vi "KundtsTube.vi"() -> ()   [LabVIEW 2015]
panel:
  in  "?":T1
  out "Gain vs Frequency":cluster{"X":dbl, "Y":dbl}[](graph)
  in  "Number of Samples":dbl
  in  "Sampling Rate":dbl
  in  "stop":bool
  out "Waveform Graph":dynamicdata(graph)
  in  "Amplitude":dbl
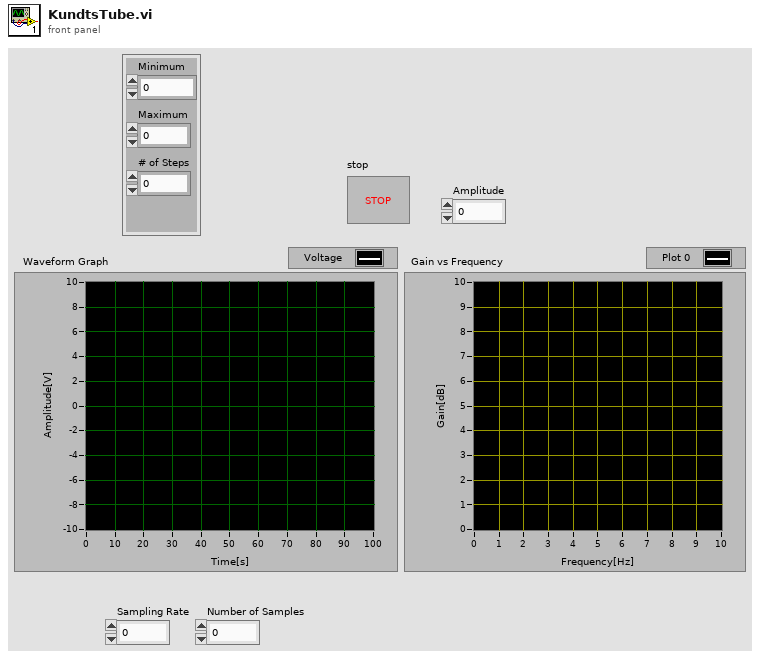
[diagram p1: front panel]
types:
  T1 = cluster{"Minimum":dbl, "Maximum":dbl, "# of Steps":dbl}
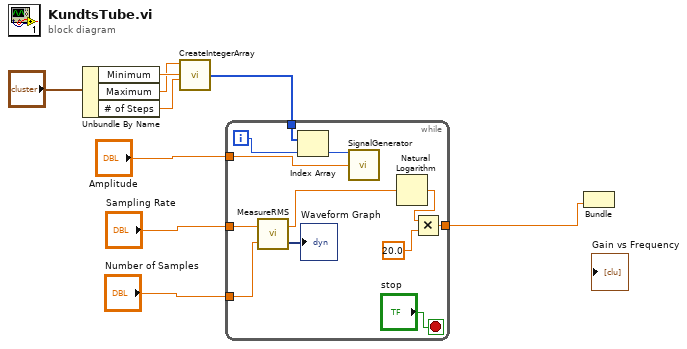
[diagram p0: block diagram]
diagram:
  n1 = Unbundle By Name("?") -> ("Minimum"=w5:dbl, "Maximum"=w4:dbl, "# of Steps"=w3:dbl)
  n2 = call "CreateIntegerArray.vi"("Number of Elements"=w3, "Minimum"=w5, "Maximum"=w4) -> ("Array"=w2:i8[])  [unwired: 1 in]
  n3 = while {
    tunnel: "Amplitude" -> [w20]
    tunnel: "Number of Samples" -> [w18]
    tunnel: "Sampling Rate" -> [w17]
    tunnel: w2 -> [w16]
    tunnel: [w10] -> w1
    i -> [w15]
    stop <- "stop" stop-if-true
    n4 = call "MeasureRMS.vi"("# of Samples"=w18, "Sampling Rate"=w17) -> ("Waveform Graph"=→"Waveform Graph":dynamicdata, "RMS"=w13:dbl)
    n5 = Index Array(array=w16, index=w15) -> (element=w14:i8)
    n6 = call "SignalGenerator.vi"("amplitude"=w20, "frequency"=w14) -> ()  [unwired: 1 in, 1 out]
    n7 = Natural Logarithm(1:w13) -> (0:w12:dbl)
    n8 = Multiply(x=w12, y=20.0) -> (x*y=w10:dbl)
  }
  n9 = Bundle(w1) -> ()  [unwired: 2 in, 1 out]
